vi "Choose File.vi"(0 "Search Directory":path=path "P:/inst/Krohn-Hite 7008/Settings", 1 "error in":errorcluster) -> (2 "Return Path":path=path "P:/inst/Krohn-Hite 7008/Settings/113885-log-3465664636.393126.ini", 3 "Loaded":bool=TRUE, 4 "error out":errorcluster)   [LabVIEW 2013]
uses:
  <vilib>/Utility/xml.llb/Read From XML File(string).vi
panel:
  in  "Tab Control":enum32{"Choose File", "Preview Settings"}(tab)
  in  "Search Pattern":string
  in  "Date":timestamp=timestamp(3466010686.4421263 s since 1904-01-01)
  in  "When":u16(ring)=2 items=["On or Before Specified", "On Specified ", "On or After Specified"]
  in  "Specific":u16(ring) items=["Specific to Month", "Specific to Day", "Specific to Hour"]
  in  "Filter by Name":bool
  in  "Filter by Date":bool
  in  "Choose":bool
  in  "Search":bool
  in  "Results":i32(listbox)
  out "Settings":T1(array[cluster])=[{"Gain"=4, "Input Coupling"=3, "Shunt Resistor"=2, "Coupling"=1, "Bandwidth Filter"=2}, {"Gain"=4, "Input Coupling"=3, "Shunt Resistor"=1, "Coupling"=2, "Bandwidth Filter"=1}, {"Gain"=2, "Input Coupling"=4, "Shunt Resistor"=2, "Coupling"=1, "Bandwidth Filter"=2}, {"Gain"=1, "Input Coupling"=1, "Shunt Resistor"=2, "Coupling"=1, "Bandwidth Filter"=2}, {"Gain"=1, "Input Coupling"=3, "Shunt Resistor"=2, "Coupling"=1, "Bandwidth Filter"=2}, {"Gain"=1, "Input Coupling"=4, "Shunt Resistor"=2, "Coupling"=1, "Bandwidth Filter"=2}, {"Gain"=3, "Input Coupling"=3, "Shunt Resistor"=2, "Coupling"=1, "Bandwidth Filter"=2}, {"Gain"=1, "Input Coupling"=4, "Shunt Resistor"=2, "Coupling"=1, "Bandwidth Filter"=2}] {"Bandwidth Filter" items=["OFF"=1, "ON"=2]; "Coupling" items=["AC"=1, "DC"=2]; "Shunt Resistor" items=["Open"=1, "50"=2, "500"=3, "5k"=4, "50k"=5]; "Input Coupling" items=["Off"=1, "SE +"=2, "SE -"=3, "Diff"=4]; "Gain" items=["1x"=1, "10x"=2, "100x"=3, "1000x"=4]}
  # "(type \"log\" to find auto-logged settings)"
  # "Input\nCoupling"
  # "Shunt\nResistor"
  # "Bandwidth\nFilter"
  # "Gain"
  # "Coupling"
  # "CH 1"
  # "CH 2"
  # "CH 3"
  # "CH 4"
  # "CH 5"
  # "CH 6"
  # "CH 7"
  # "CH 8"
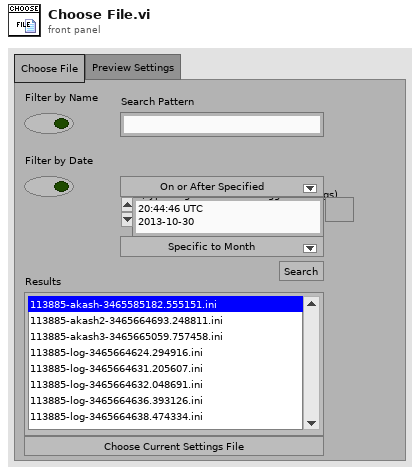
[diagram p1: front panel]
types:
  T1 = cluster{"Gain":u16, "Input Coupling":u16, "Shunt Resistor":u16, "Coupling":u16, "Bandwidth Filter":u16}[]
  T2 = typedef "LVDateTimeRec.ctl" = cluster{"fractional second":dbl, "second":i32, "minute":i32, "hour":i32, "day of month":i32, "month":i32, "year":i32, "day of week":i32, "day of year":i32, "DST":i32}
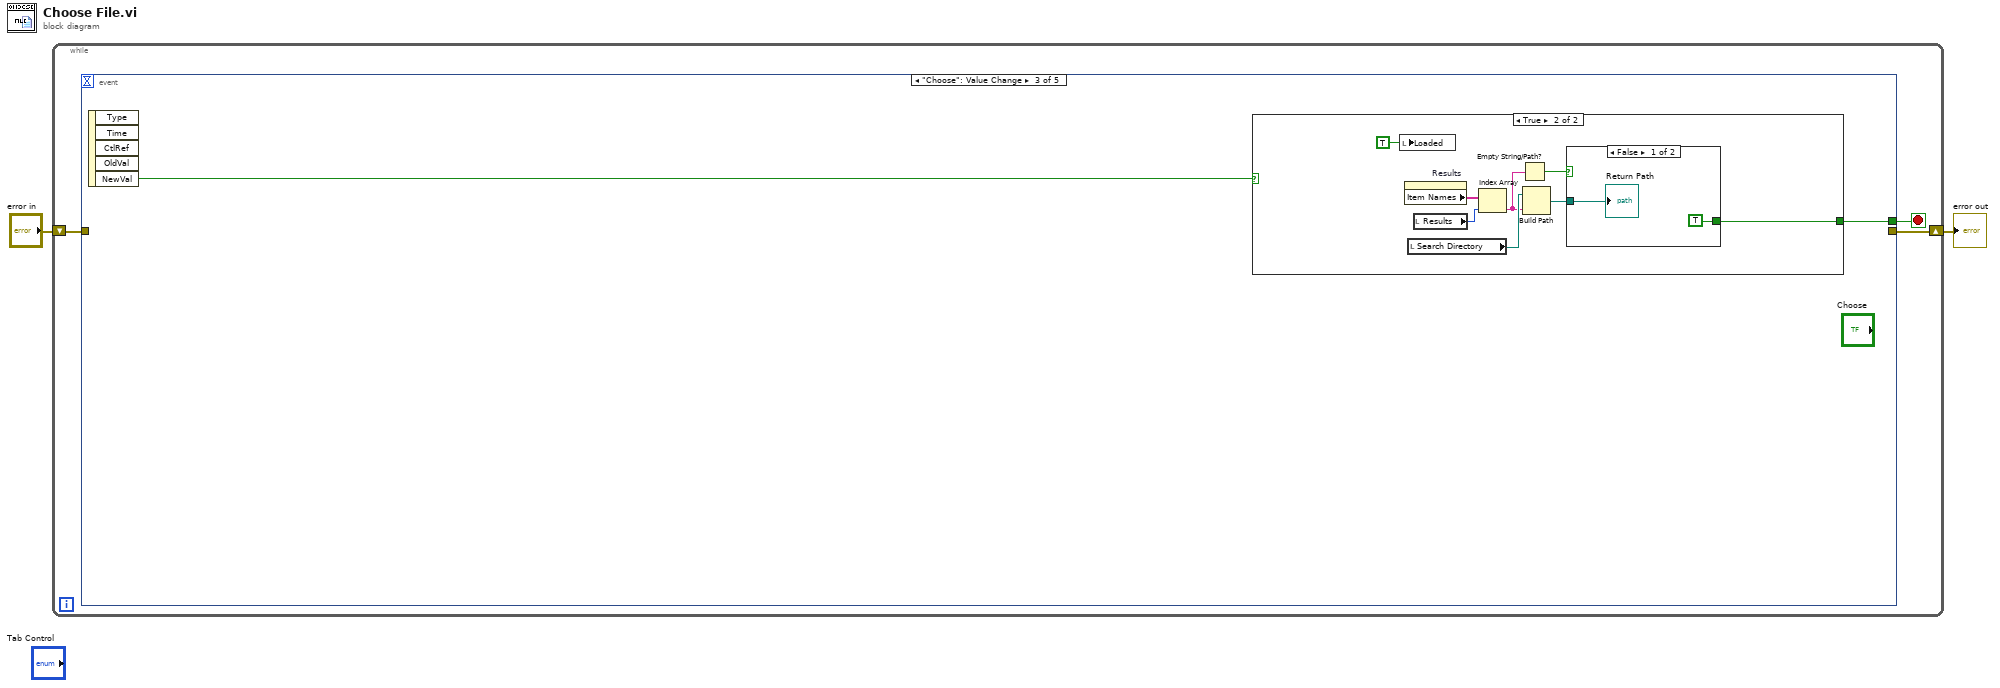
[diagram p0: block diagram]
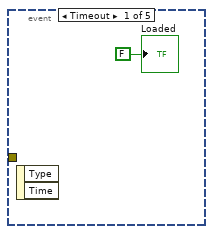
[diagram p2: hidden frame]
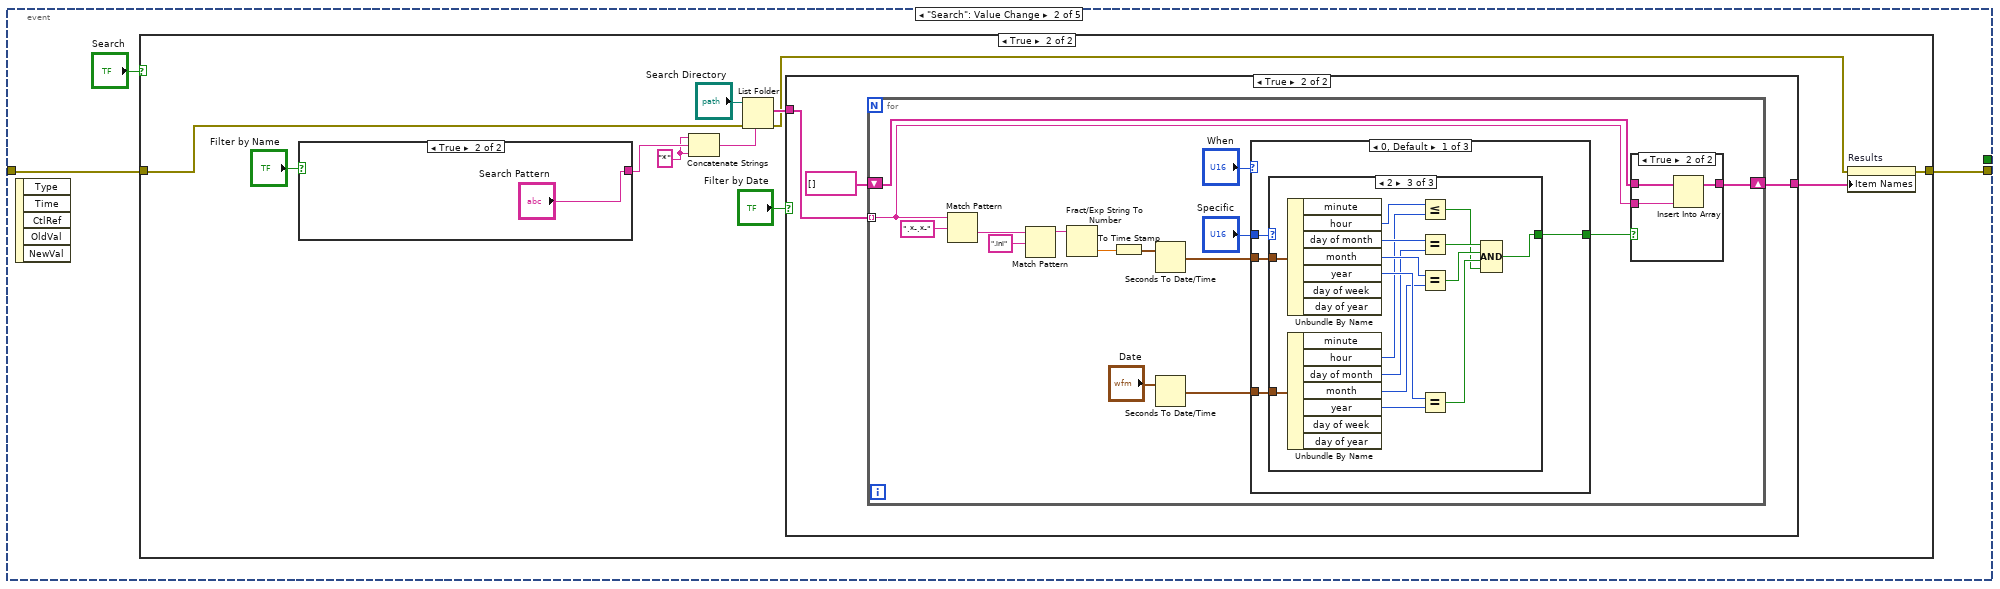
[diagram p3: hidden frame]
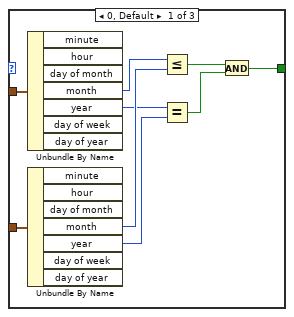
[diagram p7: hidden frame]
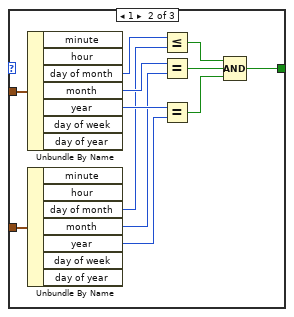
[diagram p8: hidden frame]
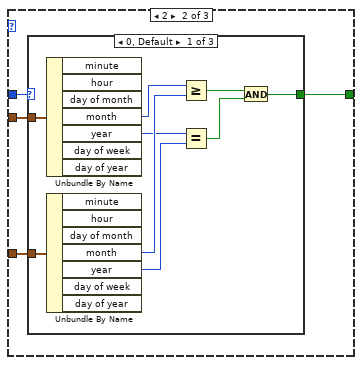
[diagram p9: hidden frame]
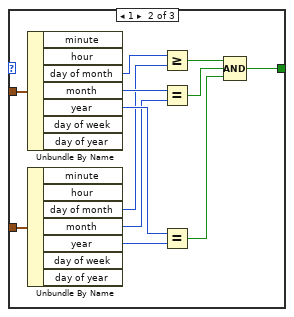
[diagram p10: hidden frame]
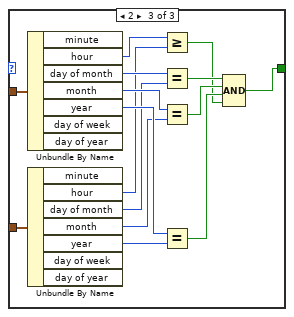
[diagram p11: hidden frame]
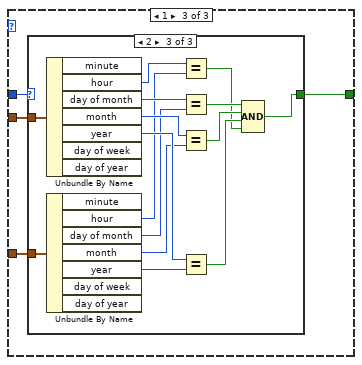
[diagram p12: hidden frame]
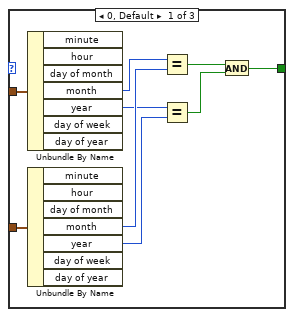
[diagram p13: hidden frame]
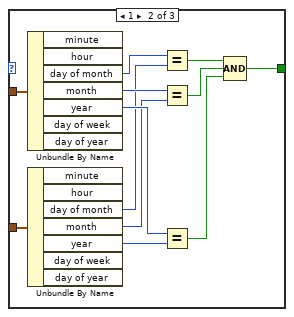
[diagram p14: hidden frame]
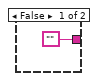
[diagram p15: hidden frame]
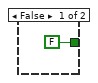
[diagram p16: hidden frame]
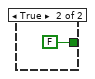
[diagram p17: hidden frame]
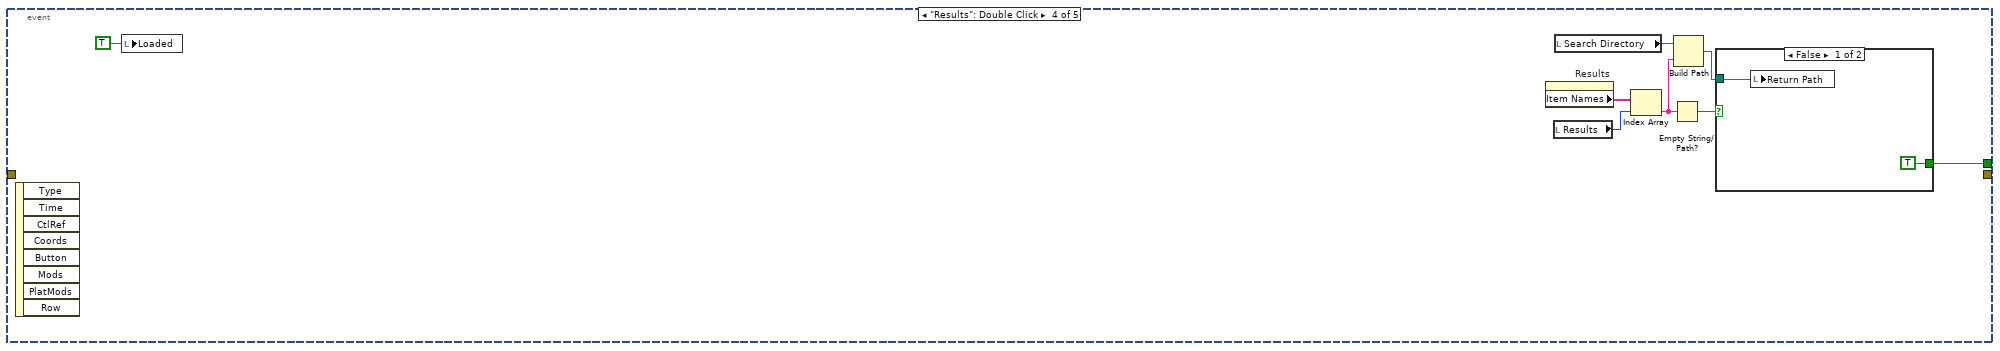
[diagram p18: hidden frame]
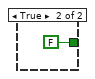
[diagram p19: hidden frame]
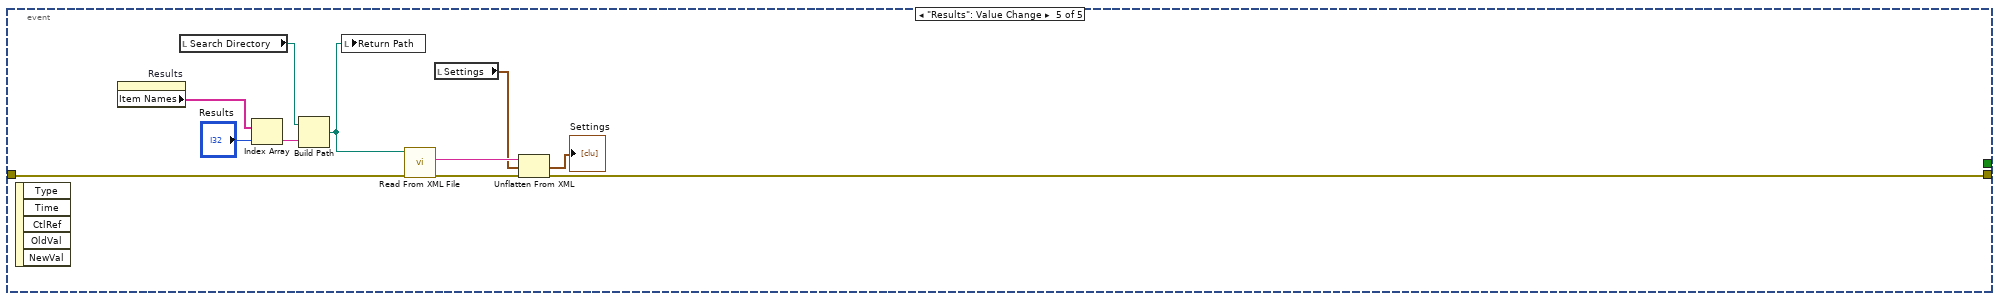
[diagram p20: hidden frame]
diagram:
  n1 = while {
    shift-right: [w5] -> w2
    shift-left: "error in" -> [w4]
    stop <- w3 stop-if-true
    n2 = event shown="[2] \"Choose\": Value Change" {
      selector: _ -> [_ _ _ _ _]
      dyn-events: _ -> [_ _ _ _ _]
      timeout: _ -> [_ _ _ _ _]
      tunnel: w4 -> [_ w8 _ _ w195]
      tunnel: [_ w7 _ _ w193] -> w5
      tunnel: [_ _ w167 w188 _] -> w3
      event Timeout {
        n3 = event-data() -> ()  [unwired: 1 in, 2 out]
        "Loaded" <- FALSE ("Loaded")
      }
      event "Search": Value Change {
        n4 = event-data() -> ()  [unwired: 1 in, 5 out]
        n5 = case shown="True" "Search" {
          tunnel: w8 -> [w10 w15]
          tunnel: [w10 w13] -> w7
          frame False {
          }
          frame True {
            w12 = "*" ("string")
            n6 = case shown="True" "Filter by Name" {
              tunnel: ["" "Search Pattern"] -> w19
              frame False {
              }
              frame True {
              }
            }
            n7 = Concatenate Strings(w12, w19, w12) -> (w11:string)
            n8 = List Folder(path="Search Directory", pattern=w11, error in=w15) -> (filenames=w17:string[], error out=w14:errorcluster)  [unwired: 1 in, 2 out]
            n9 = case shown="True" "Filter by Date" {
              tunnel: w17 -> [w22 w25]
              tunnel: [w22 w23] -> w16
              frame False {
              }
              frame True {
                n10 = for {
                  tunnel: w25 -> [w30] mode=indexing
                  shift-right: [w29] -> w23
                  shift-left: string[] [] -> [w31]
                  n11 = Match Pattern(string=w30, regular expression=".*-.*-") -> (after substring=w26:string)  [unwired: 1 in, 3 out]
                  n12 = Match Pattern(string=w26, regular expression=".ini" ("substring (\"\")")) -> (before substring=w27:string)  [unwired: 1 in, 3 out]
                  n13 = Fract/Exp String To Number(string=w27) -> (number=w37:dbl)  [unwired: 3 in, 1 out]
                  n14 = To Time Stamp(1:w37) -> (0:w36:timestamp)
                  n15 = Seconds To Date/Time(time stamp (now)=w36) -> (date time rec=w35:T2)  [unwired: 1 in]
                  n16 = Seconds To Date/Time(time stamp (now)="Date") -> (date time rec=w34:T2)  [unwired: 1 in]
                  n17 = case shown="0, Default" "When" {
                    tunnel: w35 -> [w48 w88 w128]
                    tunnel: w34 -> [w47 w87 w127]
                    tunnel: [w46 w86 w126] -> w32
                    tunnel: "Specific" -> [w45 w85 w125]
                    frame 0, Default {
                      n18 = case shown="2" w45 {
                        tunnel: w48 -> [w57 w69 w84]
                        tunnel: w47 -> [w56 w68 w83]
                        tunnel: [w49 w58 w73] -> w46
                        frame 0, Default {
                          n19 = Unbundle By Name(w57) -> ("month"=w55:i32, "year"=w52:i32)  [unwired: 5 out]
                          n20 = Unbundle By Name(w56) -> ("month"=w54:i32, "year"=w53:i32)  [unwired: 5 out]
                          n21 = Less Or Equal?(x=w55, y=w54) -> (x <= y?=w51:bool)
                          n22 = Equal?(x=w52, y=w53) -> (x = y?=w50:bool)
                          n23 = And(x=w51, y=w50) -> (x .and. y?=w49:bool)
                        }
                        frame 1 {
                          n24 = Unbundle By Name(w69) -> ("day of month"=w63:i32, "month"=w64:i32, "year"=w66:i32)  [unwired: 4 out]
                          n25 = Unbundle By Name(w68) -> ("day of month"=w62:i32, "month"=w65:i32, "year"=w67:i32)  [unwired: 4 out]
                          n26 = Less Or Equal?(x=w63, y=w62) -> (x <= y?=w61:bool)
                          n27 = Equal?(x=w64, y=w65) -> (x = y?=w60:bool)
                          n28 = Equal?(x=w66, y=w67) -> (x = y?=w59:bool)
                          n29 = Compound Arithmetic op=AND(w61, w60, w59) -> (w58:bool)
                        }
                        frame 2 {
                          n30 = Unbundle By Name(w84) -> ("hour"=w72:i32, "day of month"=w78:i32, "month"=w79:i32, "year"=w81:i32)  [unwired: 3 out]
                          n31 = Unbundle By Name(w83) -> ("hour"=w71:i32, "day of month"=w77:i32, "month"=w80:i32, "year"=w82:i32)  [unwired: 3 out]
                          n32 = Less Or Equal?(x=w72, y=w71) -> (x <= y?=w70:bool)
                          n33 = Equal?(x=w78, y=w77) -> (x = y?=w76:bool)
                          n34 = Equal?(x=w79, y=w80) -> (x = y?=w75:bool)
                          n35 = Equal?(x=w81, y=w82) -> (x = y?=w74:bool)
                          n36 = Compound Arithmetic op=AND(w76, w75, w74, w70) -> (w73:bool)
                        }
                      }
                    }
                    frame 2 {
                      n37 = case shown="0, Default" w85 {
                        tunnel: w88 -> [w97 w109 w124]
                        tunnel: w87 -> [w96 w108 w123]
                        tunnel: [w89 w98 w113] -> w86
                        frame 0, Default {
                          n38 = Unbundle By Name(w97) -> ("month"=w95:i32, "year"=w92:i32)  [unwired: 5 out]
                          n39 = Unbundle By Name(w96) -> ("month"=w94:i32, "year"=w93:i32)  [unwired: 5 out]
                          n40 = Greater Or Equal?(x=w95, y=w94) -> (x >= y?=w91:bool)
                          n41 = Equal?(x=w92, y=w93) -> (x = y?=w90:bool)
                          n42 = And(x=w91, y=w90) -> (x .and. y?=w89:bool)
                        }
                        frame 1 {
                          n43 = Unbundle By Name(w109) -> ("day of month"=w103:i32, "month"=w104:i32, "year"=w106:i32)  [unwired: 4 out]
                          n44 = Unbundle By Name(w108) -> ("day of month"=w102:i32, "month"=w105:i32, "year"=w107:i32)  [unwired: 4 out]
                          n45 = Greater Or Equal?(x=w103, y=w102) -> (x >= y?=w101:bool)
                          n46 = Equal?(x=w104, y=w105) -> (x = y?=w100:bool)
                          n47 = Equal?(x=w106, y=w107) -> (x = y?=w99:bool)
                          n48 = Compound Arithmetic op=AND(w101, w100, w99) -> (w98:bool)
                        }
                        frame 2 {
                          n49 = Unbundle By Name(w124) -> ("hour"=w112:i32, "day of month"=w118:i32, "month"=w119:i32, "year"=w121:i32)  [unwired: 3 out]
                          n50 = Unbundle By Name(w123) -> ("hour"=w111:i32, "day of month"=w117:i32, "month"=w120:i32, "year"=w122:i32)  [unwired: 3 out]
                          n51 = Greater Or Equal?(x=w112, y=w111) -> (x >= y?=w110:bool)
                          n52 = Equal?(x=w118, y=w117) -> (x = y?=w116:bool)
                          n53 = Equal?(x=w119, y=w120) -> (x = y?=w115:bool)
                          n54 = Equal?(x=w121, y=w122) -> (x = y?=w114:bool)
                          n55 = Compound Arithmetic op=AND(w116, w115, w114, w110) -> (w113:bool)
                        }
                      }
                    }
                    frame 1 {
                      n56 = case shown="2" w125 {
                        tunnel: w128 -> [w137 w149 w164]
                        tunnel: w127 -> [w136 w148 w163]
                        tunnel: [w129 w138 w153] -> w126
                        frame 0, Default {
                          n57 = Unbundle By Name(w137) -> ("month"=w135:i32, "year"=w132:i32)  [unwired: 5 out]
                          n58 = Unbundle By Name(w136) -> ("month"=w134:i32, "year"=w133:i32)  [unwired: 5 out]
                          n59 = Equal?(x=w135, y=w134) -> (x = y?=w131:bool)
                          n60 = Equal?(x=w132, y=w133) -> (x = y?=w130:bool)
                          n61 = And(x=w131, y=w130) -> (x .and. y?=w129:bool)
                        }
                        frame 1 {
                          n62 = Unbundle By Name(w149) -> ("day of month"=w143:i32, "month"=w144:i32, "year"=w146:i32)  [unwired: 4 out]
                          n63 = Unbundle By Name(w148) -> ("day of month"=w142:i32, "month"=w145:i32, "year"=w147:i32)  [unwired: 4 out]
                          n64 = Equal?(x=w143, y=w142) -> (x = y?=w141:bool)
                          n65 = Equal?(x=w144, y=w145) -> (x = y?=w140:bool)
                          n66 = Equal?(x=w146, y=w147) -> (x = y?=w139:bool)
                          n67 = Compound Arithmetic op=AND(w141, w140, w139) -> (w138:bool)
                        }
                        frame 2 {
                          n68 = Unbundle By Name(w164) -> ("hour"=w152:i32, "day of month"=w158:i32, "month"=w159:i32, "year"=w161:i32)  [unwired: 3 out]
                          n69 = Unbundle By Name(w163) -> ("hour"=w151:i32, "day of month"=w157:i32, "month"=w160:i32, "year"=w162:i32)  [unwired: 3 out]
                          n70 = Equal?(x=w152, y=w151) -> (x = y?=w150:bool)
                          n71 = Equal?(x=w158, y=w157) -> (x = y?=w156:bool)
                          n72 = Equal?(x=w159, y=w160) -> (x = y?=w155:bool)
                          n73 = Equal?(x=w161, y=w162) -> (x = y?=w154:bool)
                          n74 = Compound Arithmetic op=AND(w156, w155, w154, w150) -> (w153:bool)
                        }
                      }
                    }
                  }
                  n75 = case shown="True" w32 {
                    tunnel: w31 -> [w41 w44]
                    tunnel: w30 -> [_ w43]
                    tunnel: [w41 w42] -> w29
                    frame False {
                    }
                    frame True {
                      n76 = Insert Into Array(array=w44, new element=w43) -> (w42:string[])  [unwired: 1 in]
                    }
                  }
                }
              }
            }
            n77 = property on="Results" class="LstBox (strict)"(error in=w14, "Item Names"=w16) -> (error out=w13:errorcluster)  [unwired: 1 in, 1 out]
          }
        }
      }
      event "Choose": Value Change {
        n78 = event-data() -> ("NewVal"=w168:bool)  [unwired: 1 in, 4 out]
        n79 = case shown="True" w168 {
          tunnel: [FALSE w170] -> w167
          frame False {
          }
          frame True {
            n80 = local write "Loaded"(TRUE ("Loaded")) -> ()
            n81 = property on="Results" class="LstBox (strict)"() -> ("Item Names"=w177:string[])  [unwired: 2 in, 2 out]
            n82 = local read "Search Directory"() -> (w176:path)
            n83 = local read "Results"() -> (w174:i32)
            n84 = Index Array(array=w177, index=w174) -> (element=w172:string)
            n85 = Empty String/Path?(string/path=w172) -> (empty?=w171:bool)
            n86 = Build Path(base path=w176, name or relative path=w172) -> (appended path=w175:path)
            n87 = case shown="False" w171 {
              tunnel: w175 -> [w179 _]
              tunnel: [TRUE FALSE] -> w170
              frame False {
                "Return Path" <- w179
              }
              frame True {
              }
            }
          }
        }
      }
      event "Results": Double Click {
        n88 = event-data() -> ()  [unwired: 1 in, 8 out]
        n89 = local write "Loaded"(TRUE ("Loaded")) -> ()
        n90 = property on="Results" class="LstBox (strict)"() -> ("Item Names"=w187:string[])  [unwired: 2 in, 2 out]
        n91 = local read "Results"() -> (w184:i32)
        n92 = local read "Search Directory"() -> (w186:path)
        n93 = Index Array(array=w187, index=w184) -> (element=w182:string)
        n94 = Empty String/Path?(string/path=w182) -> (empty?=w181:bool)
        n95 = Build Path(base path=w186, name or relative path=w182) -> (appended path=w185:path)
        n96 = case shown="False" w181 {
          tunnel: w185 -> [w189 _]
          tunnel: [TRUE FALSE] -> w188
          frame False {
            n97 = local write "Return Path"(w189) -> ()
          }
          frame True {
          }
        }
      }
      event "Results": Value Change {
        n98 = event-data() -> ()  [unwired: 1 in, 5 out]
        n99 = property on="Results" class="LstBox (strict)"() -> ("Item Names"=w202:string[])  [unwired: 2 in, 2 out]
        n100 = local read "Search Directory"() -> (w201:path)
        n101 = Index Array(array=w202, index="Results") -> (element=w200:string)
        n102 = Build Path(base path=w201, name or relative path=w200) -> (appended path=w192:path)
        n103 = local write "Return Path"(w192) -> ()
        n104 = call-poly <vilib>:"Read From XML File.vi"("error in (no error)"=w195, "XML File Path"=w192) -> ("error out"=w194:errorcluster, "XML Elements"=w198:string)  [unwired: 7 in, 1 out]
        n105 = local read "Settings"() -> (w197:T1)
        n106 = Unflatten From XML(xml string=w198, type=w197, error in (no error)=w194) -> (value=→"Settings":T1, error out=w193:errorcluster)
      }
    }
  }
  "error out" <- w2
